vi "Rohde & Schwarz VNA Set Start and Stop Frequencies.vi"(6 "Channel":i8=1 min=1 max=99 step=1, 7 "Rohde & Schwarz VNA":T1, 8 "error in (no error)":errorcluster, 9 "CW? (f)":bool, 10 "Start/Stop Freqs, MHz":cluster{"Fstart":dbl, "Fstop":dbl}, 11 "VISA Resource Name":refnum<visa-resource-name>) -> (0 "error out":errorcluster, 3 "dup VISA Resource Name":refnum<visa-resource-name>)   [LabVIEW 2011]
doc: "This VI for the HP 8753B is used to read the number of stimulus points."
uses:
  TypeDefs/Rohde & Schwarz VNA Instrument Info.ctl
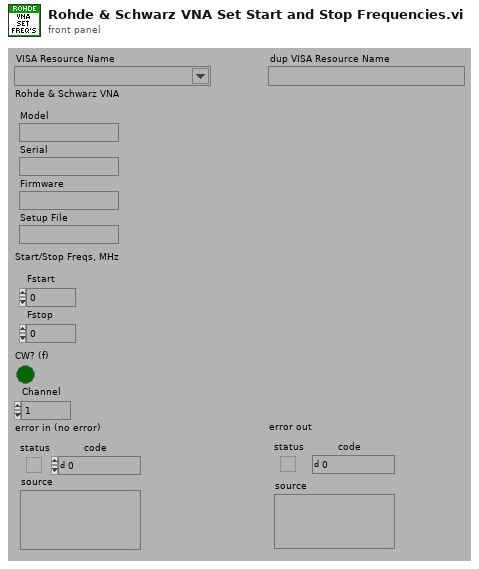
[diagram p1: front panel]
types:
  T1 = typedef "Rohde & Schwarz VNA Instrument Info.ctl" = cluster{"Model":string, "Serial":string, "Firmware":string, "Setup File":string}
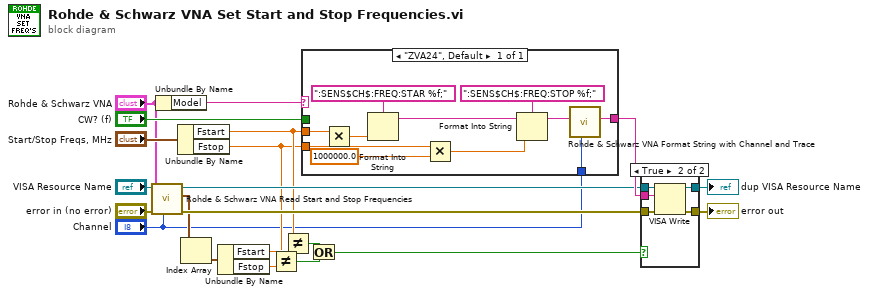
[diagram p0: block diagram]
diagram:
  n1 = call "Rohde & Schwarz VNA Read Start and Stop Frequencies.vi"("Channel"="Channel", "Rohde & Schwarz VNA"="Rohde & Schwarz VNA", "error in (no error)"="error in (no error)", "VISA Resource Name"="VISA Resource Name") -> ("error out"=w14:errorcluster, "Start/Stop Freqs, MHz"=w12:cluster{"Fstart":dbl, "Fstop":dbl}[], "dup VISA Resource Name"=w13:refnum<visa-resource-name>)  [unwired: 5 out]
  n2 = Unbundle By Name("Rohde & Schwarz VNA") -> ("Model"=w1:string)
  n3 = Unbundle By Name("Start/Stop Freqs, MHz") -> ("Fstart"=w10:dbl, "Fstop"=w8:dbl)
  n4 = Index Array(array=w12) -> (element=w11:cluster{"Fstart":dbl, "Fstop":dbl})  [unwired: 1 in]
  n5 = Unbundle By Name(w11) -> ("Fstart"=w9:dbl, "Fstop"=w7:dbl)
  n6 = Not Equal?(x=w8, y=w7) -> (x != y?=w5:bool)
  n7 = Not Equal?(x=w10, y=w9) -> (x != y?=w6:bool)
  n8 = case shown="\"ZVA24\", Default" w1 {
    tunnel: [w23] -> w18
    tunnel: "CW? (f)" -> [_]
    tunnel: w10 -> [w29]
    tunnel: w8 -> [w27]
    tunnel: "Channel" -> [w22]
    frame "ZVA24", Default {
      w25 = 1000000.0 ("y")
      n9 = Multiply(x=w29, y=w25) -> (x*y=w28:dbl)
      n10 = Format Into String(format string=":SENS$CH$:FREQ:STAR %f;", w28) -> (resulting string=w30:string)  [unwired: 2 in, 1 out]
      n11 = Multiply(x=w27, y=w25) -> (x*y=w26:dbl)
      n12 = Format Into String(format string=":SENS$CH$:FREQ:STOP %f;", initial string=w30, w26) -> (resulting string=w24:string)  [unwired: 1 in, 1 out]
      n13 = call "Rohde & Schwarz VNA Format String with Channel and Trace.vi"("Channel"=w22, "String"=w24) -> ("String Out"=w23:string)  [unwired: 1 in, 6 out]
    }
  }
  n14 = Or(x=w6, y=w5) -> (x .or. y?=w4:bool)
  n15 = case shown="True" w4 {
    tunnel: [w34 w39] -> w21
    tunnel: [w33 w38] -> w20
    tunnel: w18 -> [_ w37]
    tunnel: w14 -> [w33 w36]
    tunnel: w13 -> [w34 w35]
    frame False {
    }
    frame True {
      n16 = VISA Write(VISA resource name=w35, write buffer=w37, error in (no error)=w36) -> (VISA resource name out=w39:refnum<visa-resource-name>, error out=w38:errorcluster)  [unwired: 1 out]
    }
  }
  "dup VISA Resource Name" <- w21
  "error out" <- w20
